vi "Get Sub-Entry.vi"(8 "Error In":errorcluster, 10 "Sub-Index":u8 format="%.0x", 11 "reference in":refnum<class "OD Entry.lvclass">) -> (0 "Error Out":errorcluster, 1 "Found?":bool, 2 "OD Sub-Entry":refnum<class "OD Sub-Entry.lvclass">, 3 "reference out":refnum<class "OD Entry.lvclass">)   [LabVIEW 2019, in "Electronic Datasheet.lvlib" / "OD Entry.lvclass"]
uses:
  OD Entry.lvclass
  OD Sub-Entry/OD Sub-Entry.lvclass
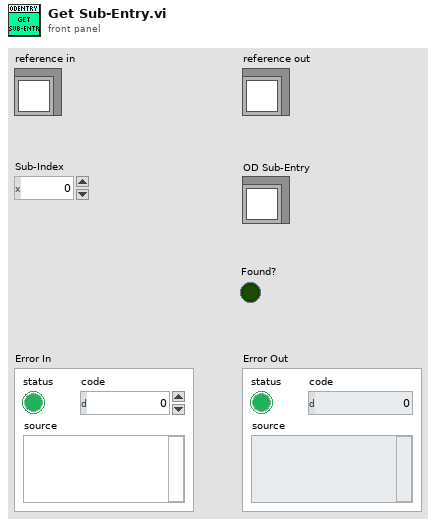
[diagram p1: front panel]
types:
  T1 = typedef "Electronic Datasheet.lvlib/OD Entry.lvclass/ObjectAttributes.ctl" = cluster{"Index":u16, "ObjectType":refnum<class "Object Type Base.lvclass">, "Denotation":string, "Count":u8, "ObjExtend":u8, "Label":string, "Description":string, "PDO Mapping Type":T2, "Sub-Entries":map{u8, refnum<class "OD Sub-Entry.lvclass">}}
  T2 = typedef "Electronic Datasheet.lvlib/PDO Mapping Type.ctl" = enum16{"no", "optional", "RPDO", "TPDO", "UNKNOWN"}
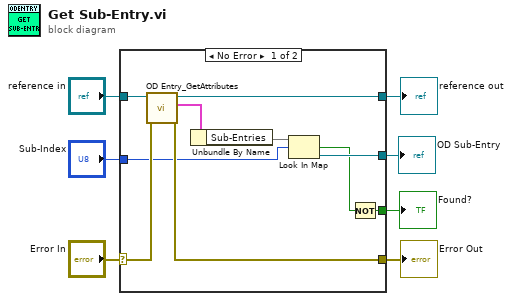
[diagram p0: block diagram]
diagram:
  n1 = case shown="No Error" "Error In" {
    selector: "Error In" -> [w17 w19]
    tunnel: [w15 w19] -> w6
    tunnel: [w13 w18] -> w4
    tunnel: "reference in" -> [w14 w18]
    tunnel: "Sub-Index" -> [w11 _]
    tunnel: [w10 _] -> w2
    tunnel: [w8 _] -> w1
    frame No Error {
      n2 = call "OD Entry_GetAttributes.vi"("Error In"=w17, "reference in"=w14) -> ("Error Out"=w15:errorcluster, "Data"=w16:T1, "reference out"=w13:refnum<class "OD Entry.lvclass">)  [unwired: 6 in, 1 out]
      n3 = Unbundle By Name(w16) -> ("Sub-Entries"=w12:map{u8, refnum<class "OD Sub-Entry.lvclass">})
      n4 = Look In Map(map=w12, key=w11) -> (key not found?=w9:bool, value=w10:refnum<class "OD Sub-Entry.lvclass">)  [unwired: 1 in]
      n5 = Not(x=w9) -> (.not. x?=w8:bool)
    }
    frame Error {
    }
  }
  "Error Out" <- w6
  "reference out" <- w4
  "OD Sub-Entry" <- w2
  "Found?" <- w1
